vi "DAQ Channel Array to ExperimentStateCluster.vi"(8 "First Trigger Time":dbl, 9 "DAQ Channel Array":T2 {"Card Settings"."Start Time" format="%#_6f"; "Card Settings"."End Time" format="%#_6f"; "Card Settings"."Rate" format="%#_6p"}, 11 "Experiment State":T1={"Send Trigger 3"=FALSE, "error"={"status"=FALSE, "code"=0, "source"=""}, "Digitizer DAQmx Tasks"={"TaskArray"=[]}, "Digitizer Settings"={"6133 Digitizer Channels"=[], "Global Edge Type"=10280, "Total Samples"=[], "Pre-Trigger Samples"=[], "Sample Rate"=[], "Trigger Sources"=[], "Voltage Ranges"=[], "Channel Names"=[], "Active"=[], "Samples to remove"=[], "Start Time"=[], "End Time"=[]}, "Synchronization Settings"={"Synchronizer"="PXI1Slot2", "source terminal"="GlobalSoftwareTrigger"}, "Digitizer Data"=[], "Next Shot#"="0", "System Message"="", "User Shot Notes"="", "Timing Settings"={"Timing Card Settings"=[], "Timing Channel Settings"=[[{"Delay (s)"=2.559999942779541, "Pulse width (s)"=0.009999999776482582, "Active"=TRUE, "Channel Name"="Fiber 8", "counter"="PXI1Slot8/ctr7"}]]}} {"Timing Settings"."Timing Channel Settings"."Pulse width (s)" format="%.3p"; "Timing Settings"."Timing Channel Settings"."Delay (s)" format="%.3p"; "Digitizer Settings"."Sample Rate" format="%#_3p"; "Digitizer Settings"."Global Edge Type" items=["Rising"=10280, "Falling"=10171]}) -> (3 "Experiment State Out":T1={"Send Trigger 3"=FALSE, "error"={"status"=FALSE, "code"=0, "source"=""}, "Digitizer DAQmx Tasks"={"TaskArray"=[]}, "Digitizer Settings"={"6133 Digitizer Channels"=[], "Global Edge Type"=10280, "Total Samples"=[], "Pre-Trigger Samples"=[], "Sample Rate"=[], "Trigger Sources"=[], "Voltage Ranges"=[], "Channel Names"=[], "Active"=[], "Samples to remove"=[], "Start Time"=[], "End Time"=[]}, "Synchronization Settings"={"Synchronizer"="PXI1Slot2", "source terminal"="GlobalSoftwareTrigger"}, "Digitizer Data"=[], "Next Shot#"="0", "System Message"="", "User Shot Notes"="", "Timing Settings"={"Timing Card Settings"=[], "Timing Channel Settings"=[[{"Delay (s)"=2.559999942779541, "Pulse width (s)"=0.009999999776482582, "Active"=TRUE, "Channel Name"="Fiber 8", "counter"="PXI1Slot8/ctr7"}]]}} {"Timing Settings"."Timing Channel Settings"."Pulse width (s)" format="%.3p"; "Timing Settings"."Timing Channel Settings"."Delay (s)" format="%.3p"; "Digitizer Settings"."Sample Rate" format="%#_3p"; "Digitizer Settings"."Global Edge Type" items=["Rising"=10280, "Falling"=10171]})   [LabVIEW 2013]
doc: "Converts DAQ Channel Array information to Experiment State Cluster format.\n\nOnly takes the first active Trigger from DAQ card array"
uses:
  Controls/DAQ Channel Array.ctl
  Controls/DAQ Card Channel Array.ctl
  Controls/DAQ Card Settings.ctl
  Controls/ExperimentStateCluster.ctl
panel:
  # "Channel Settings"
  # "Card Wide Settings"
  # "Channel Settings"
  # "Card Wide Settings"
  # "Channel                                     Name                                                               Voltage Range                    Card Settings"
  # "Sampling Rate [1/s]"
  # "Start Time [s]"
  # "End Time [s]"
  # "Slot"
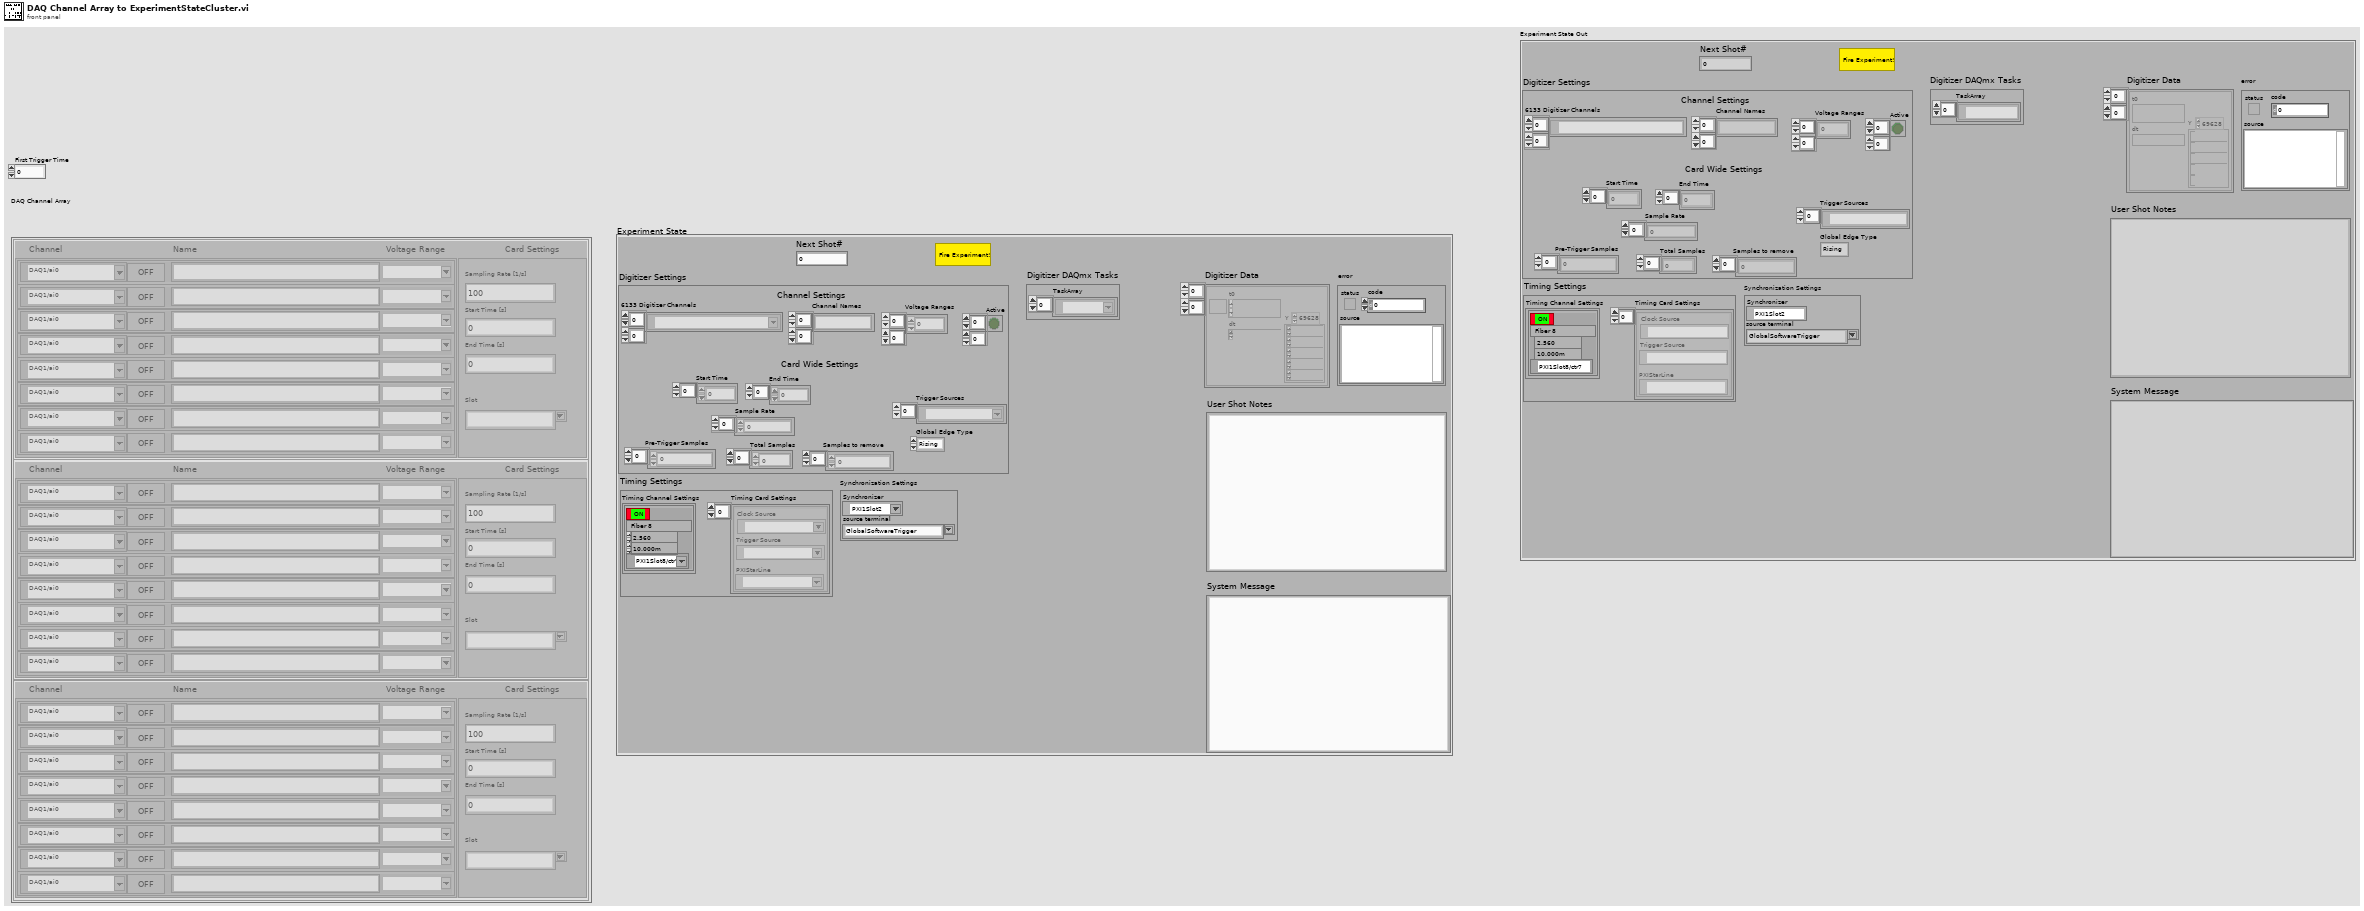
[diagram p1: front panel]
types:
  T1 = typedef "ExperimentStateCluster.ctl" = cluster{"Send Trigger 3":bool, "error":errorcluster, "Digitizer DAQmx Tasks":cluster{"TaskArray":refnum<k21>[]}, "Digitizer Settings":cluster{"6133 Digitizer Channels":tag[][], "Global Edge Type":i32, "Total Samples":i32[], "Pre-Trigger Samples":u32[], "Sample Rate":dbl[], "Trigger Sources":tag[], "Voltage Ranges":dbl[][], "Channel Names":string[][], "Active":bool[][], "Samples to remove":u32[], "Start Time":dbl[], "End Time":dbl[]}, "Synchronization Settings":cluster{"Synchronizer":refnum<k15>, "source terminal":string}, "Digitizer Data":waveform(dbl)[][], "Next Shot#":string, "System Message":string, "User Shot Notes":string, "Timing Settings":cluster{"Timing Card Settings":cluster{"Trigger Source":tag, "Clock Source":tag, "PXIStarLine":tag}[], "Timing Channel Settings":cluster{"Delay (s)":dbl, "Pulse width (s)":dbl, "Active":bool, "Channel Name":string, "counter":tag}[][]}}
  T2 = typedef "DAQ Channel Array.ctl" = cluster{"DAQ Channel Array":T3, "Card Settings":T4}[]
  T3 = typedef "DAQ Card Channel Array.ctl" = cluster{"Active":bool, "Channel Name":string, "Channel":tag, "Voltage Range":string}[]
  T4 = typedef "DAQ Card Settings.ctl" = cluster{"Rate":dbl, "End Time":dbl, "Start Time":dbl, "SlotTrigger":string}
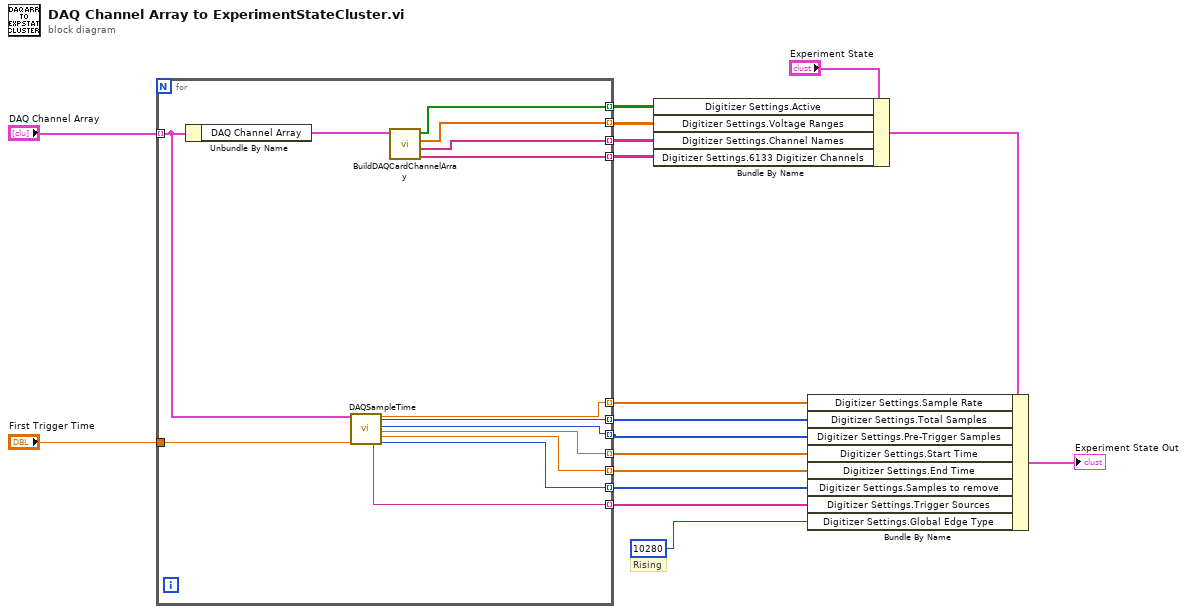
[diagram p0: block diagram]
diagram:
  # "Rising"
  n1 = for {
    tunnel: "DAQ Channel Array" -> [w26] mode=indexing
    tunnel: [w29] -> w12 mode=indexing
    tunnel: [w28] -> w13 mode=indexing
    tunnel: [w27] -> w14 mode=indexing
    tunnel: [w30] -> w15 mode=indexing
    tunnel: "First Trigger Time" -> [w25]
    tunnel: [w24] -> w10 mode=indexing
    tunnel: [w23] -> w9 mode=indexing
    tunnel: [w22] -> w8 mode=indexing
    tunnel: [w21] -> w7 mode=indexing
    tunnel: [w20] -> w5 mode=indexing
    tunnel: [w19] -> w4 mode=indexing
    tunnel: [w18] -> w3 mode=indexing
    n2 = Unbundle By Name(w26) -> ("DAQ Channel Array"=w31:T3)
    n3 = call "DAQSampleTime.vi"("Cluster"=w26, "First Trigger Time"=w25) -> ("SlotTrigger"=w21:string, "Rate"=w24:dbl, "Total Samples"=w23:i32, "Pre-trigger Samples"=w22:i32, "Start Time"=w18:dbl, "End Time"=w19:dbl, "Samples to remove"=w20:i32)  [unwired: 11 in]
    n4 = call "BuildDAQCardChannelArray.vi"("DAQ Channel Array"=w31) -> ("Channel"=w27:tag[], "Channel Name"=w28:string[], "Voltage Range"=w29:dbl[], "Active"=w30:bool[])  [unwired: 7 in]
  }
  n5 = Bundle By Name(cluster="Experiment State", "Digitizer Settings.Active"=w15, "Digitizer Settings.Voltage Ranges"=w12, "Digitizer Settings.Channel Names"=w13, "Digitizer Settings.6133 Digitizer Channels"=w14) -> (w6:T1)
  n6 = Bundle By Name(cluster=w6, "Digitizer Settings.Sample Rate"=w10, "Digitizer Settings.Total Samples"=w9, "Digitizer Settings.Pre-Trigger Samples"=w8, "Digitizer Settings.Start Time"=w3, "Digitizer Settings.End Time"=w4, "Digitizer Settings.Samples to remove"=w5, "Digitizer Settings.Trigger Sources"=w7, "Digitizer Settings.Global Edge Type"=10280 ("Channels.Edge Type")) -> (→"Experiment State Out":T1)
